vi "Globales Snake.vi"() -> ()   [LabVIEW 2021, in "Game.lvclass"]
uses:
  Game.lvclass
panel:
  in  "Playing Time":u32
  in  "player name":string
  out "Stop Back Music":bool
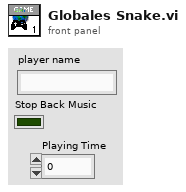
[diagram p1: front panel]
diagram:
